vi "Add Slot JSON to Base JSON.vi"(8 "error in (no error)":errorcluster, 9 "Slot Topology Variant":variant, 11 "Base Topology Variant":variant) -> (0 "error out":errorcluster, 3 "Base Topology Variant out":variant)   [LabVIEW 2017]
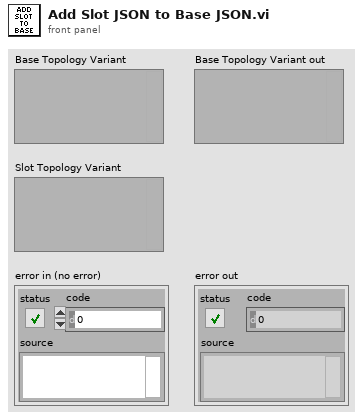
[diagram p1: front panel]
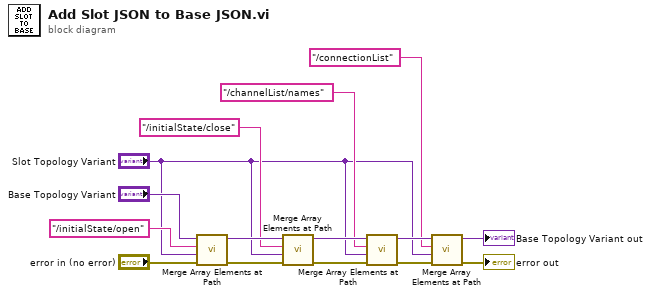
[diagram p0: block diagram]
diagram:
  n1 = call "Merge Array Elements at Path.vi"("error in (no error)"="error in (no error)", "Slot Topology Variant"="Slot Topology Variant", "Path String"="/initialState/open", "Base Topology Variant"="Base Topology Variant") -> ("error out"=w12:errorcluster, "Base Topology Variant out"=w10:variant)  [unwired: 6 in]
  n2 = call "Merge Array Elements at Path.vi"("error in (no error)"=w12, "Slot Topology Variant"="Slot Topology Variant", "Path String"="/initialState/close", "Base Topology Variant"=w10) -> ("error out"=w11:errorcluster, "Base Topology Variant out"=w7:variant)  [unwired: 6 in]
  n3 = call "Merge Array Elements at Path.vi"("error in (no error)"=w11, "Slot Topology Variant"="Slot Topology Variant", "Path String"="/channelList/names", "Base Topology Variant"=w7) -> ("error out"=w8:errorcluster, "Base Topology Variant out"=w5:variant)  [unwired: 6 in]
  n4 = call "Merge Array Elements at Path.vi"("error in (no error)"=w8, "Slot Topology Variant"="Slot Topology Variant", "Path String"="/connectionList", "Base Topology Variant"=w5) -> ("error out"=→"error out":errorcluster, "Base Topology Variant out"=→"Base Topology Variant out":variant)  [unwired: 6 in]
